vi "niDTS BT INSTR RX Configure BT Header.vi"(8 "error in (no error)":errorcluster, 11 "niDTS BT INSTR RX in":refnum<class "niDTS BT INSTR RX.lvclass">) -> (0 "error out":errorcluster, 3 "niDTS BT INSTR RX out":refnum<class "niDTS BT INSTR RX.lvclass">)   [LabVIEW 2015, in "niDTS BT.lvlib" / "niDTS BT INSTR RX.lvclass"]
uses:
  niDTS BT INSTR RX.lvclass
  niDTS BT INSTR RX.lvclass/niDTS BT INSTR RX.ctl
  RiviInstDriver/niRfsgBT/Objects/niRfsgBt.lvclass
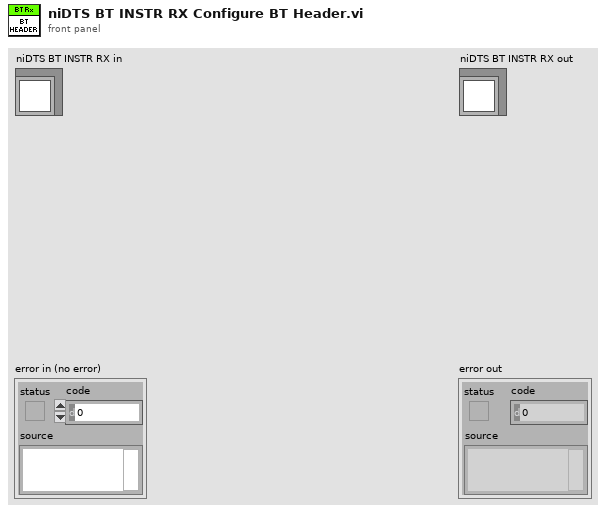
[diagram p1: front panel]
types:
  T1 = cluster{"HeaderLTAddress":i32, "HeaderFlowControlBit":bool, "ArqnBit":enum16{"NAK", "ACK"}, "SeqnBit":bool}
  T2 = typedef "niRfsgBT.lvclass/niRfsgBT INC Handle.ctl" = refnum<data-value>
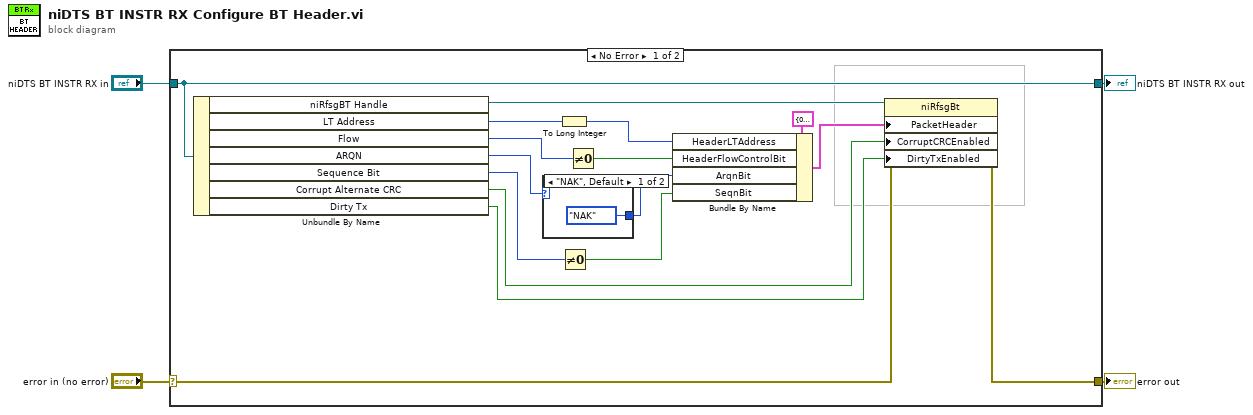
[diagram p0: block diagram]
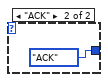
[diagram p2: hidden frame]
diagram:
  n1 = case shown="No Error" "error in (no error)" {
    selector: "error in (no error)" -> [w9 w24]
    tunnel: [w8 w24] -> w3
    tunnel: [w20 w23] -> w1
    tunnel: "niDTS BT INSTR RX in" -> [w20 w23]
    frame No Error {
      n2 = Unbundle By Name(w20) -> ("niRfsgBT Handle"=w19:T2, "LT Address"=w16:i8, "Flow"=w15:i8, "ARQN"=w12:enum16{"NAK", "ACK"}, "Sequence Bit"=w10:i8, "Corrupt Alternate CRC"=w6:bool, "Dirty Tx"=w5:bool)
      n3 = case shown="\"NAK\", Default" w12 {
        tunnel: [enum16{"NAK", "ACK"}."NAK" ("ArqnBit") enum16{"NAK", "ACK"}."ACK" ("ArqnBit")] -> w13
        frame "NAK", Default {
        }
        frame "ACK" {
        }
      }
      n4 = To Long Integer(number=w16) -> (32bit integer=w17:i32)
      n5 = Not Equal To 0?(x=w10) -> (x != 0?=w11:bool)
      n6 = Not Equal To 0?(x=w15) -> (x != 0?=w14:bool)
      n7 = Bundle By Name(cluster=T1 {"HeaderLTAddress"=0, "HeaderFlowControlBit"=FALSE, "ArqnBit"=enum."NAK", "SeqnBit"=FALSE} ("SOURce:RFSG:BLUetooth:PACKet:HEADer"), "HeaderLTAddress"=w17, "HeaderFlowControlBit"=w14, "ArqnBit"=w13, "SeqnBit"=w11) -> (w7:T1)
      n8 = property class="niRfsgBt"(reference=w19, error in=w9, "PacketHeader"=w7, "CorruptCRCEnabled"=w6, "DirtyTxEnabled"=w5) -> (error out=w8:errorcluster)  [unwired: 1 out]
    }
    frame Error {
    }
  }
  "error out" <- w3
  "niDTS BT INSTR RX out" <- w1
